vi "UE_master_Create.vi"(8 "error in (no error)":errorcluster, 9 "Command UE":refnum<user-event>, 10 "ID":string, 11 "reference in":refnum<class "UE_master.lvclass">) -> (0 "error out":errorcluster, 3 "reference out":refnum<class "UE_master.lvclass">)   [LabVIEW 2019, in "CommandResponse communication.lvlib" / "UE_master.lvclass"]
doc: "Constructor."
uses:
  UE_master.lvclass
  C:/Program Files/National Instruments/LabVIEW 2019/vi.lib/addons/_AddQ/G#Object/G#Object.lvclass
  C:/Barkhausen mmWave radar/Development/LV/Barkhausen mmWave hardware control/Host/Intertarget communication/CR_master_class/CR_master.lvclass
  Command + data + response cluster.ctl
  Status + response + data cluster.ctl
  <vilib>/addons/_AddQ/G#Object/G#Object.lvclass
  CR_master_class/CR_master.lvclass
  CommandResponse communication.lvlib
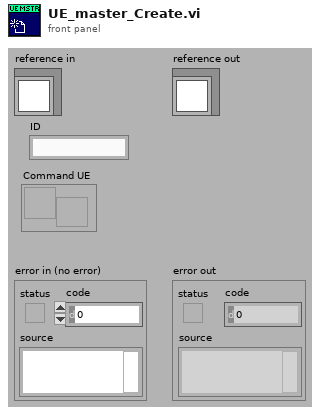
[diagram p1: front panel]
types:
  T1 = typedef "CommandResponse communication.lvlib/UE_master.lvclass/ObjectAttributesRef.ctl" = refnum<data-value>
  T2 = typedef "CommandResponse communication.lvlib/UE_master.lvclass/ObjectAttributes.ctl" = cluster{"Command UE":refnum<user-event>}
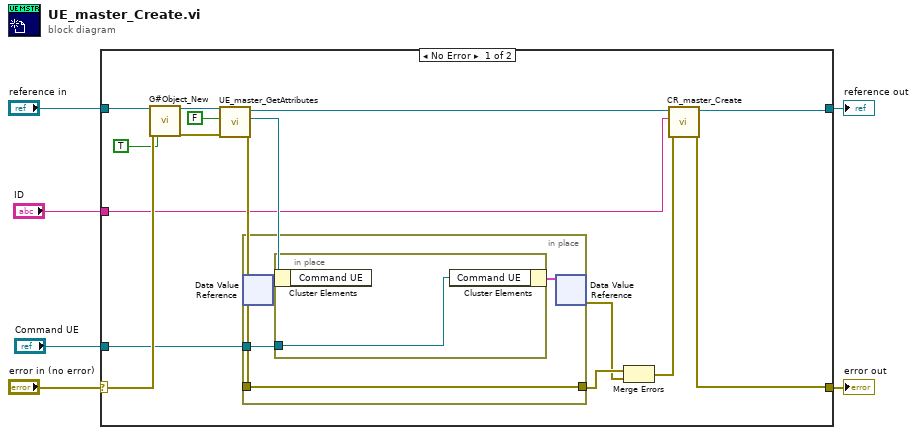
[diagram p0: block diagram]
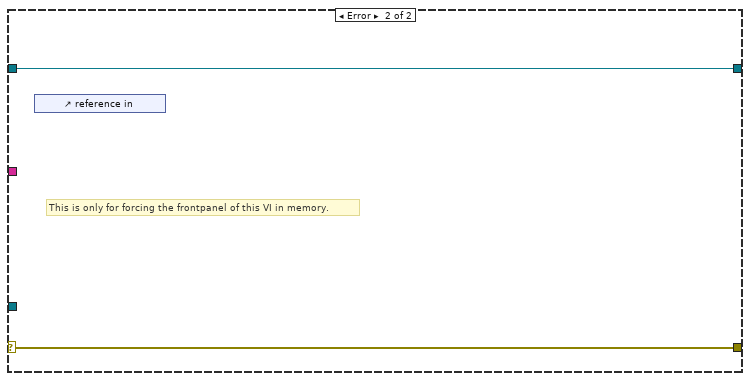
[diagram p2: hidden frame]
diagram:
  n1 = case shown="No Error" "error in (no error)" {
    selector: "error in (no error)" -> [w21 w29]
    tunnel: [w9 w29] -> w5
    tunnel: [w11 w28] -> w3
    tunnel: "reference in" -> [w22 w28]
    tunnel: "Command UE" -> [w8 _]
    tunnel: "ID" -> [w7 _]
    frame No Error {
      n2 = call <vilib>:"G#Object_New.vi"("reference in"=w22, "error in (no error)"=w21, "user counter (T)?"=TRUE ("User Counter")) -> ("reference out"=w14:refnum<class "UE_master.lvclass">, "error out"=w13:errorcluster)  [unwired: 14 in, 1 out]
      n3 = call "UE_master_GetAttributes.vi"("error in (no error)"=w13, "return data? (T)"=FALSE ("return data"), "reference in"=w14) -> ("error out"=w17:errorcluster, "attributes ref"=w16:T1, "reference out"=w12:refnum<class "UE_master.lvclass">)  [unwired: 5 in, 1 out]
      n4 = in-place {
        in-place-border: w17 -> [w24]
        in-place-border: [w24] -> w19
        in-place-border: w8 -> [w23]
        n5 = in-place-dvr #1(w16) -> (w25:T2)  [unwired: 1 out]
        n6 = in-place {
          in-place-border: w23 -> [w27]
          n7 = in-place-cluster #2(w25) -> ()  [unwired: 1 out]
          n8 = in-place-cluster #2("Command UE"=w27) -> (w26:T2)
        }
        n9 = in-place-dvr #1(w26) -> (w18:errorcluster)  [unwired: 1 out]
      }
      n10 = Merge Errors(w19, w18) -> (w10:errorcluster)
      n11 = call "CR_master_Create.vi"("error in (no error)"=w10, "ID"=w7, "reference in"=w12) -> ("error out"=w9:errorcluster, "reference out"=w11:refnum<class "UE_master.lvclass">)  [unwired: 7 in]
    }
    frame Error {
      # "This is only for forcing the frontpanel of this VI in memory."
      n12 = control-ref of="reference in"() -> ()  [unwired: 1 out]
    }
  }
  "error out" <- w5
  "reference out" <- w3
